vi "MAX31855USB_open.vi"(8 "error in (no error)":errorcluster, 9 "Serial Configuration":T1={"Baud Rate"=9600, "Parity"=0, "Data Bits"=8, "Stop Bits"=10, "Flow Control"=0} {"Flow Control" items=["None", "XON/XOFF", "RTS/CTS", "XON/XOFF & RTS/CTS", "DTR/DSR", "XON/XOFF & DTR/DSR"]; "Stop Bits" items=["1.0"=10, "1.5"=15, "2.0"=20]; "Data Bits" items=["7"=7, "8"=8]; "Parity" items=["None", "Odd", "Even", "Mark", "Space"]; "Baud Rate" items=["300"=300, "600"=600, "1200"=1200, "2400"=2400, "4800"=4800, "9600"=9600, "19200"=19200]}, 10 "ID Query (True)":bool=TRUE, 11 "VISA resource name":refnum<visa-resource-name>) -> (0 "error out":errorcluster, 3 "VISA resource name out":refnum<visa-resource-name>)   [LabVIEW 2014]
uses:
  <vilib>/Instr/_visa.llb/VISA Configure Serial Port (Instr).vi
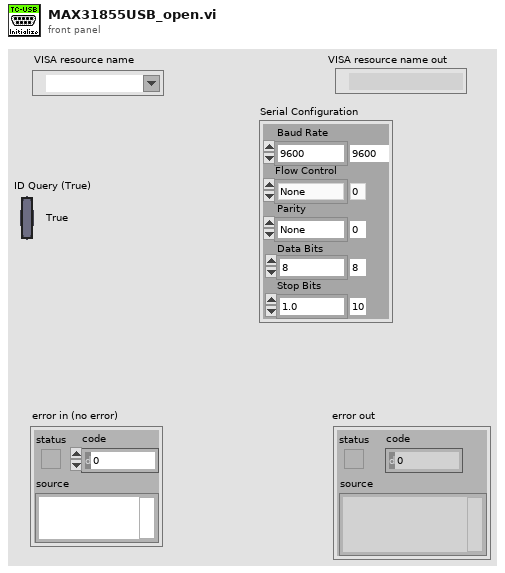
[diagram p1: front panel]
types:
  T1 = cluster{"Baud Rate":u32, "Parity":u16, "Data Bits":u16, "Stop Bits":u16, "Flow Control":u16}
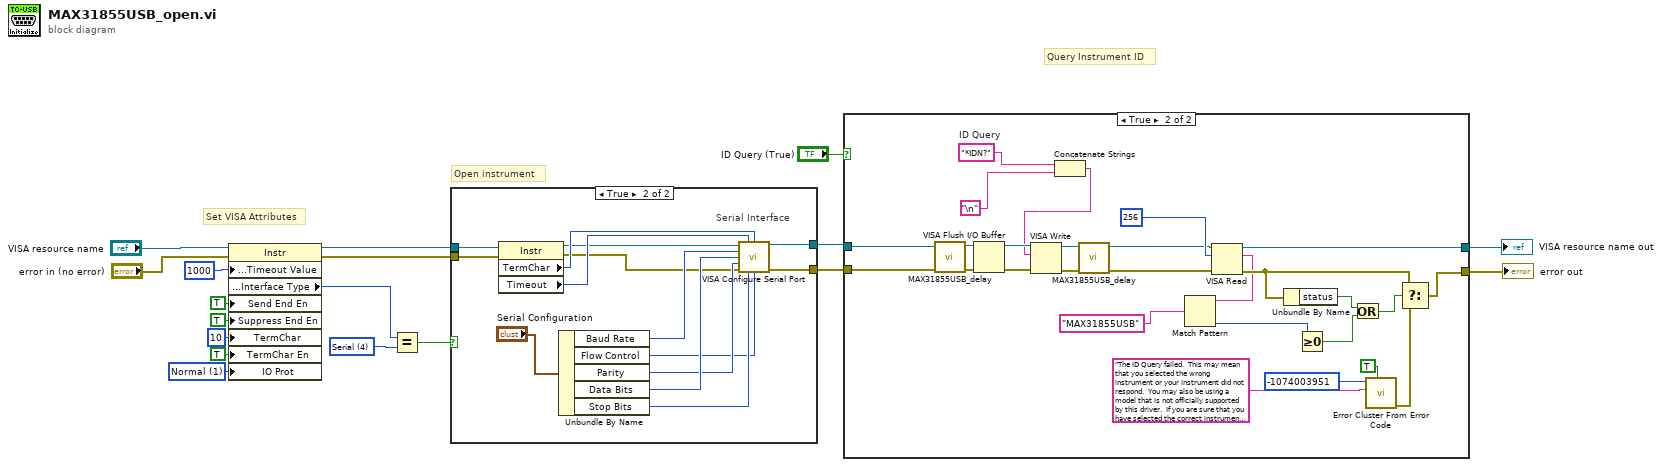
[diagram p0: block diagram]
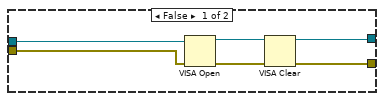
[diagram p2: hidden frame]
diagram:
  w8 = u16 1 items=["Normal"=1, "VXI/FDC"=2, "GPIB/HS488"=3, "Serial-TCPIP-USB/488 Strings"=4, "USBTMC/Vendor-Specific"=5] ("Message Based Settings:IO Protocol")
  w13 = u16 4 items=["GPIB"=1, "VXI"=2, "GPIB-VXI"=3, "Serial"=4, "PXI"=5, "TCPIP"=6, "USB"=7] ("Interface Information:Interface Type")
  # "Set VISA Attributes"
  # "Query Instrument ID"
  # "Open instrument"
  n1 = property class="Instr"(reference="VISA resource name", error in="error in (no error)", "General Settings:Timeout Value"=u32 1000, "Send End En"=TRUE ("Message Based Settings:Send End Enable"), "Suppress End En"=TRUE ("Message Based Settings:Suppress End Enable"), "TermChar"=u8 10 ("Message Based Settings:Termination Character"), "TermChar En"=TRUE ("Message Based Settings:Termination Character Enable"), "IO Prot"=w8) -> (reference out=w16:refnum<visa-resource-name>, error out=w15:errorcluster, "Interface Information:Interface Type"=w17:u16)
  n2 = Equal?(x=w17, y=w13) -> (x = y?=w14:bool)
  n3 = case shown="True" w14 {
    tunnel: [w21 w26] -> w5
    tunnel: [w19 w25] -> w4
    tunnel: w16 -> [w24 w32]
    tunnel: w15 -> [w23 w31]
    frame False {
      n4 = VISA Open(error in (no error)=w23, VISA resource name=w24) -> (VISA resource name=w22:refnum<visa-resource-name>, error out=w20:errorcluster)  [unwired: 3 in]
      n5 = VISA Clear(VISA resource name=w22, error in (no error)=w20) -> (VISA resource name out=w21:refnum<visa-resource-name>, error out=w19:errorcluster)
    }
    frame True {
      # "Serial Interface"
      n6 = property class="Instr"(reference=w32, error in=w31) -> (reference out=w27:refnum<visa-resource-name>, error out=w28:errorcluster, "TermChar"=w30:u8, "Timeout"=w29:u32)
      n7 = Unbundle By Name("Serial Configuration") -> ("Baud Rate"=w37:u32, "Flow Control"=w33:u16, "Parity"=w35:u16, "Data Bits"=w36:u16, "Stop Bits"=w34:u16)
      n8 = call-poly "VISA Configure Serial Port"("VISA resource name"=w27, "timeout (10sec)"=w29, "termination char\n(0xA = '\\n' = LF)"=w30, "baud rate (9600)"=w37, "data bits (8)"=w36, "parity (0:none)"=w35, "error in (no error)"=w28, "stop bits (10: 1 bit)"=w34, "flow control (0:none)"=w33) -> ("VISA resource name out"=w26:refnum<visa-resource-name>, "error out"=w25:errorcluster)  [unwired: 5 in]
    }
  }
  n9 = case shown="True" "ID Query (True)" {
    tunnel: [w39 w67] -> w2
    tunnel: [w40 w66] -> w3
    tunnel: w5 -> [w40 w47]
    tunnel: w4 -> [w39 w46]
    frame False {
    }
    frame True {
      w45 = "*IDN?"  # ID Query
      n10 = call "MAX31855USB_delay.vi"("error in (no error)"=w46, "VISA Refnum in"=w47) -> ("error out"=w49:errorcluster, "VISA Refnum out"=w48:refnum<visa-resource-name>)  [unwired: 8 in]
      n11 = VISA Flush I/O Buffer(VISA resource name=w48, error in (no error)=w49) -> (VISA resource name out=w51:refnum<visa-resource-name>, error out=w50:errorcluster)  [unwired: 1 in]
      n12 = Concatenate Strings(w45, "\n") -> (w44:string)
      n13 = VISA Write(VISA resource name=w51, write buffer=w44, error in (no error)=w50) -> (VISA resource name out=w54:refnum<visa-resource-name>, error out=w53:errorcluster)  [unwired: 1 out]
      n14 = call "MAX31855USB_delay.vi"("error in (no error)"=w53, "VISA Refnum in"=w54) -> ("error out"=w41:errorcluster, "VISA Refnum out"=w42:refnum<visa-resource-name>)  [unwired: 8 in]
      n15 = VISA Read(VISA resource name=w42, byte count=u32 256, error in (no error)=w41) -> (VISA resource name out=w66:refnum<visa-resource-name>, read buffer=w55:string, error out=w60:errorcluster)  [unwired: 1 out]
      n16 = Match Pattern(string=w55, regular expression="MAX31855USB" ("read buffer")) -> (offset past match=w61:i32)  [unwired: 1 in, 3 out]
      n17 = Unbundle By Name(w60) -> ("status"=w59:bool)
      n18 = Greater Or Equal To 0?(x=w61) -> (x >= 0?=w58:bool)
      n19 = Or(x=w59, y=w58) -> (x .or. y?=w57:bool)
      n20 = call <vilib>:"Error Cluster From Error Code.vi"("show call chain? (False)"=TRUE, "error message (\"\")"="The ID Query failed.  This may mean that you selected the wrong instrument or your instrument did not respond.  You may also be using a model that is not officially supported by this driver.  If you are sure that you have selected the correct instrument and it is responding, try disabling the ID Query." ("Source (VI Name)"), "error code (0)"=-1074003951 ("Code")) -> ("error out"=w65:errorcluster)  [unwired: 6 in]
      n21 = Select(t=w60, s=w57, f=w65) -> (s? t:f=w67:errorcluster)
    }
  }
  "VISA resource name out" <- w3
  "error out" <- w2
